vi "HVACmotesTemperature.vi"() -> ()   [LabVIEW 2011]
uses:
  <vilib>/picture/picture.llb/Draw True-Color Pixmap.vi
panel:
  out "Node ID":u8
  out "Temperature":dbl(graph)
  in  "header size":i32=9
  in  "bytes to read":i32=10
  out "Packet Payload":string
  in  "Enable Read":bool=TRUE
  in  "Port Number":i32=9002
  out "KTH  Automatic Control \nTemplates. Read from SerialForwarder":picture
  # "For TestSerialCommMsg:\nheaderSize = 9\npayload = 10"
  # "Communication control"
  # "Communication results"
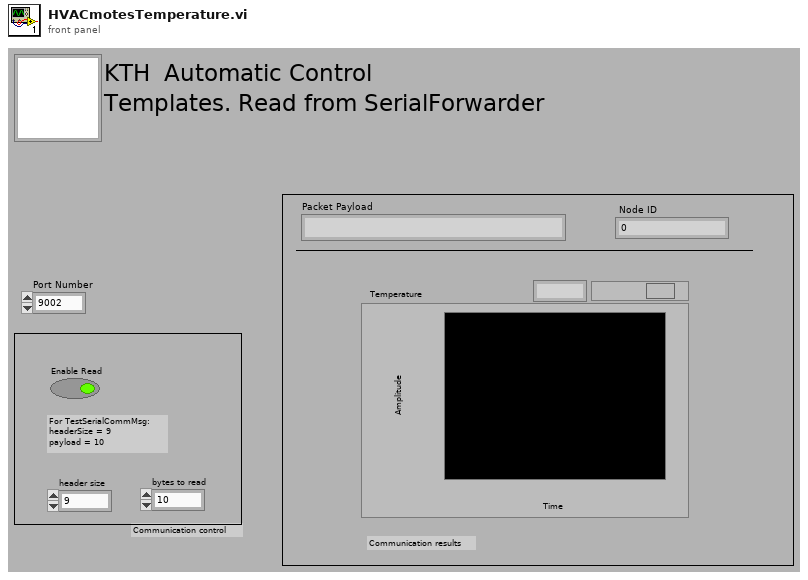
[diagram p1: front panel]
types:
  T1 = enum16{"open", "replace", "create", "open or create", "replace or create", "replace or create with confirmation"}
  T2 = typedef "imagedata.ctl" = cluster{"image type":i32, "image depth":i32, "image":u8[], "mask":u8[], "colors":u32[], "Rectangle":cluster{"left":i16, "top":i16, "right":i16, "bottom":i16}}
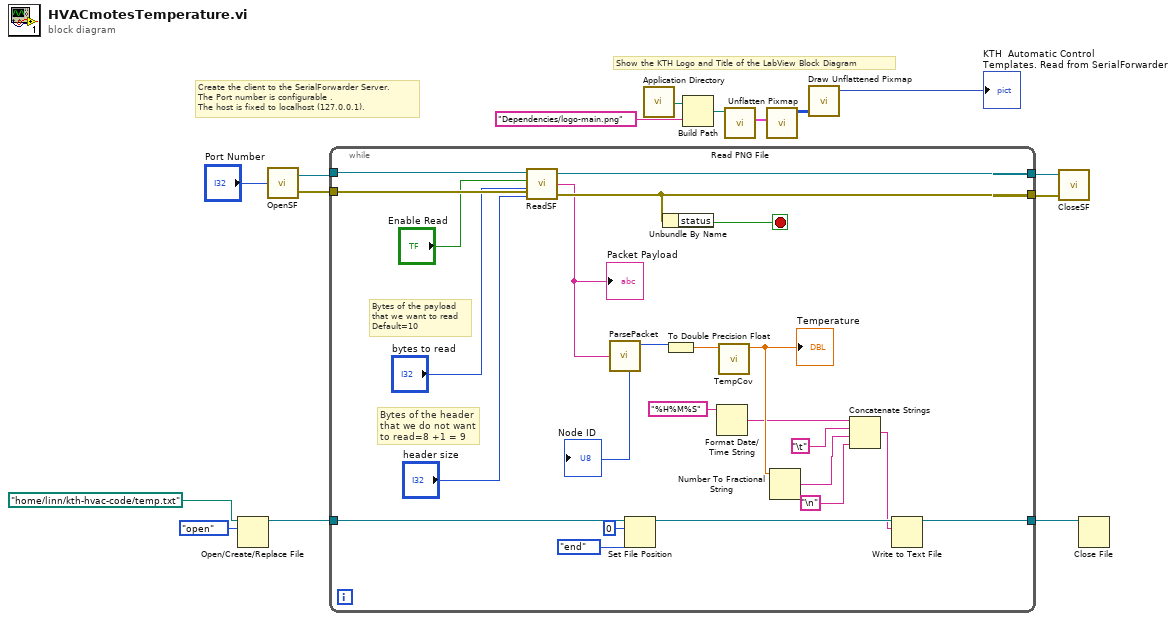
[diagram p0: block diagram]
diagram:
  # "Create the client to the SerialForwarder Server.\nThe Port number is configurable . \nThe host is fixed to localhost (127.0.0.1)."
  # "Show the KTH Logo and Title of the LabView Block Diagram"
  n1 = Open/Create/Replace File(file path (use dialog)=path "/home/linn/kth-hvac-code/temp.txt" ("file (use dialog)"), operation (0:open)=T1."open") -> (refnum out=w2:refnum<file>)  [unwired: 4 in, 2 out]
  n2 = call "OpenSF.vi"("Port Number"="Port Number") -> ("error out"=w14:errorcluster, "connection ID"=w15:refnum<k5>)
  n3 = while {
    tunnel: w15 -> [w38]
    tunnel: w14 -> [w39]
    tunnel: [w37] -> w13
    tunnel: [w35] -> w12
    tunnel: w2 -> [w24]
    tunnel: [w25] -> w1
    stop <- w36 stop-if-true
    # "Bytes of the payload \nthat we want to read\nDefault=10"
    # "Bytes of the header\nthat we do not want \nto read=8 +1 = 9"
    n4 = call "ReadSF.vi"("connection ID in"=w38, "error in"=w39, "enabled"="Enable Read", "bytes to read"="bytes to read", "header size"="header size") -> ("connection ID out"=w37:refnum<k5>, "string"=w31:string, "error out"=w35:errorcluster)  [unwired: 1 in]
    "Packet Payload" <- w31
    n5 = call "ParsePacket.vi"("data out"=w31) -> ("Node ID"=→"Node ID":u8, "Temperature"=w30:u16)  [unwired: 4 out]
    n6 = Set File Position(offset (in bytes) (0)=i64 0, refnum=w24, from (0:start)=enum16{"start", "end", "current"}."end") -> (refnum out=w21:refnum<file>)  [unwired: 1 in, 1 out]
    n7 = Unbundle By Name(w35) -> ("status"=w36:bool)
    n8 = To Double Precision Float(number=w30) -> (double precision float=w29:dbl)
    n9 = Format Date/Time String(time format string (%c)="%H%M%S") -> (date/time string=w20:string)  [unwired: 2 in]
    n10 = call "TempCov.vi"("Input x"=w29) -> ("Temperature"=w26:dbl)  [unwired: 10 in]
    "Temperature" <- w26
    n11 = Number To Fractional String(number=w26) -> (F-format string=w19:string)  [unwired: 3 in]
    n12 = Concatenate Strings(w20, "\t", w19, "\n") -> (w18:string)
    n13 = Write to Text File(file (use dialog)=w21, text=w18) -> (refnum out=w25:refnum<file>)  [unwired: 2 in, 2 out]
  }
  n14 = call <vilib>:"Application Directory.vi"() -> ("Application Directory"=w7:path)
  n15 = Build Path(base path=w7, name or relative path="Dependencies/logo-main.png") -> (appended path=w8:path)
  n16 = call <vilib>:"Read PNG File.vi"("path to PNG file"=w8) -> ("image data"=w11:T2)  [unwired: 8 in, 2 out]
  n17 = call <vilib>:"Unflatten Pixmap.vi"("image data"=w11) -> ("24-bit pixmap"=w10:u32[][])  [unwired: 4 in, 6 out]
  n18 = call-poly <vilib>:"Draw Unflattened Pixmap.vi"("data (RGB format)"=w10) -> ("new picture"=→"KTH  Automatic Control \nTemplates. Read from SerialForwarder":picture)  [unwired: 8 in]
  n19 = call "CloseSF.vi"("error out"=w12, "connection ID"=w13) -> ()  [unwired: 1 in]
  n20 = Close File(refnum=w1) -> ()  [unwired: 1 in, 2 out]
